vi "OnOff Read.vi"(8 "error in":errorcluster, 11 "Chiller in":refnum<class "Chiller.lvclass">) -> (0 "error out":errorcluster, 1 "Changed or First Call?":bool, 2 "OnOff ACT":bool, 3 "Chiller out":refnum<class "Chiller.lvclass">)   [LabVIEW 2023, in "Chiller.lvclass"]
uses:
  Chiller.lvclass
  Chiller.lvclass/Chiller.ctl
  Low Level Capabilities/OnOff/OnOff.lvclass
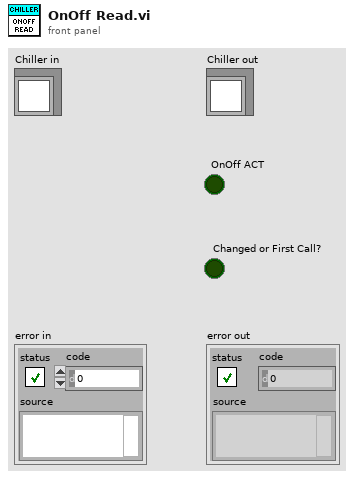
[diagram p1: front panel]
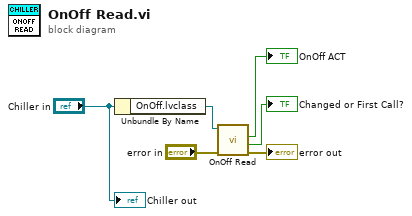
[diagram p0: block diagram]
diagram:
  n1 = Unbundle By Name("Chiller in") -> ("OnOff.lvclass"=w6:refnum<class "OnOff.lvclass">)
  n2 = call-dynamic "OnOff Read.vi"("error in"="error in", "OnOff in"=w6) -> ("error out"=→"error out":errorcluster, "Changed or First Call?"=→"Changed or First Call?":bool, "OnOff ACT"=→"OnOff ACT":bool)  [unwired: 6 in, 1 out]
  "Chiller out" <- "Chiller in"
